vi "Analyze L1,L2,L3 states.vi"(8 "error in":errorcluster, 11 "read buffer":string) -> (0 "error out":errorcluster, 2 "Result":bool, 3 "LED state":dbl)   [LabVIEW 2020]
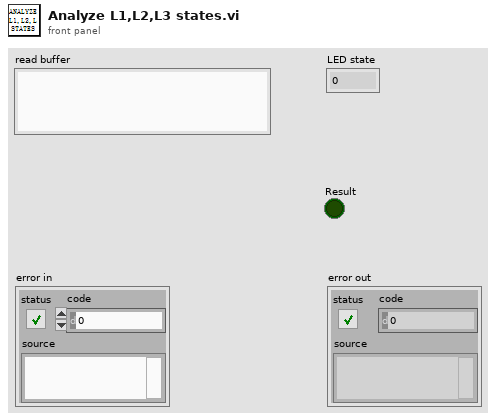
[diagram p1: front panel]
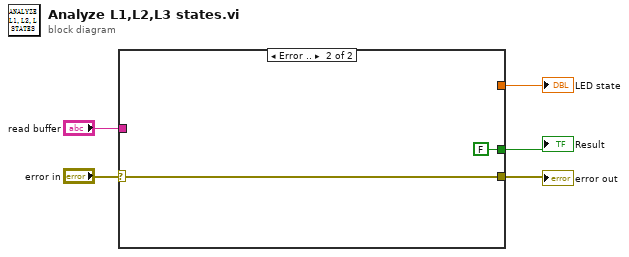
[diagram p0: block diagram]
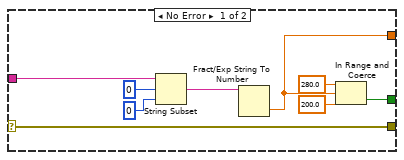
[diagram p2: hidden frame]
diagram:
  n1 = case shown="Error .." "error in" {
    selector: "error in" -> [w10 w16]
    tunnel: "read buffer" -> [w14 _]
    tunnel: [w9 _] -> w4
    tunnel: [w10 w16] -> w2
    tunnel: [w6 FALSE] -> w1
    frame No Error {
      n2 = String Subset(string=w14, offset (0)=0, length (rest)=0 ("length (rest)")) -> (substring=w11:string)
      n3 = Fract/Exp String To Number(string=w11) -> (number=w9:dbl)  [unwired: 3 in, 1 out]
      n4 = In Range and Coerce(upper limit=280.0, x=w9, lower limit=200.0) -> (In Range?=w6:bool)  [unwired: 1 out]
    }
    frame Error {
    }
  }
  "LED state" <- w4
  "error out" <- w2
  "Result" <- w1
